vi "超标留样通讯.vi"(8 "error in (no error)":errorcluster, 9 "VISA resource name":refnum<visa-resource-name> caption="VISA资源名称", 10 "写入缓冲区":string, 11 "功能输入":enum16{"打开串口", "写入", "读取", "关闭串口"}(ring)) -> (0 "error out":errorcluster, 2 "读取缓冲区":string, 3 "VISA resource name out":refnum<visa-resource-name>)   [LabVIEW 2016, in "超标留样集成.lvlib" / "德润DR803M超标留样.lvlib"]
uses:
  <vilib>/Instr/_visa.llb/VISA Configure Serial Port (Instr).vi
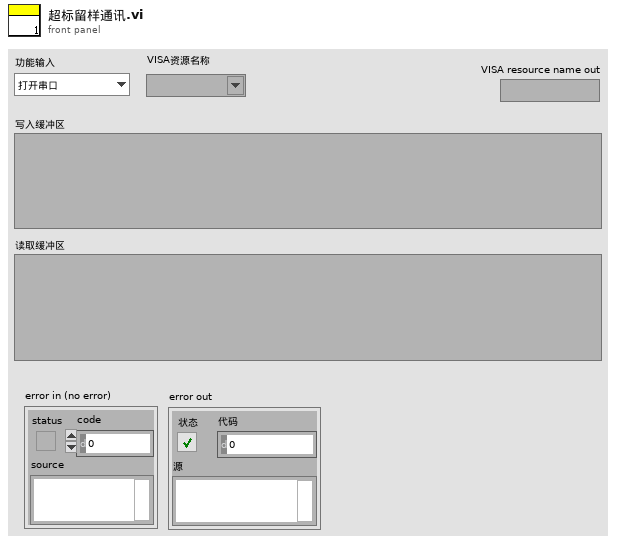
[diagram p1: front panel]
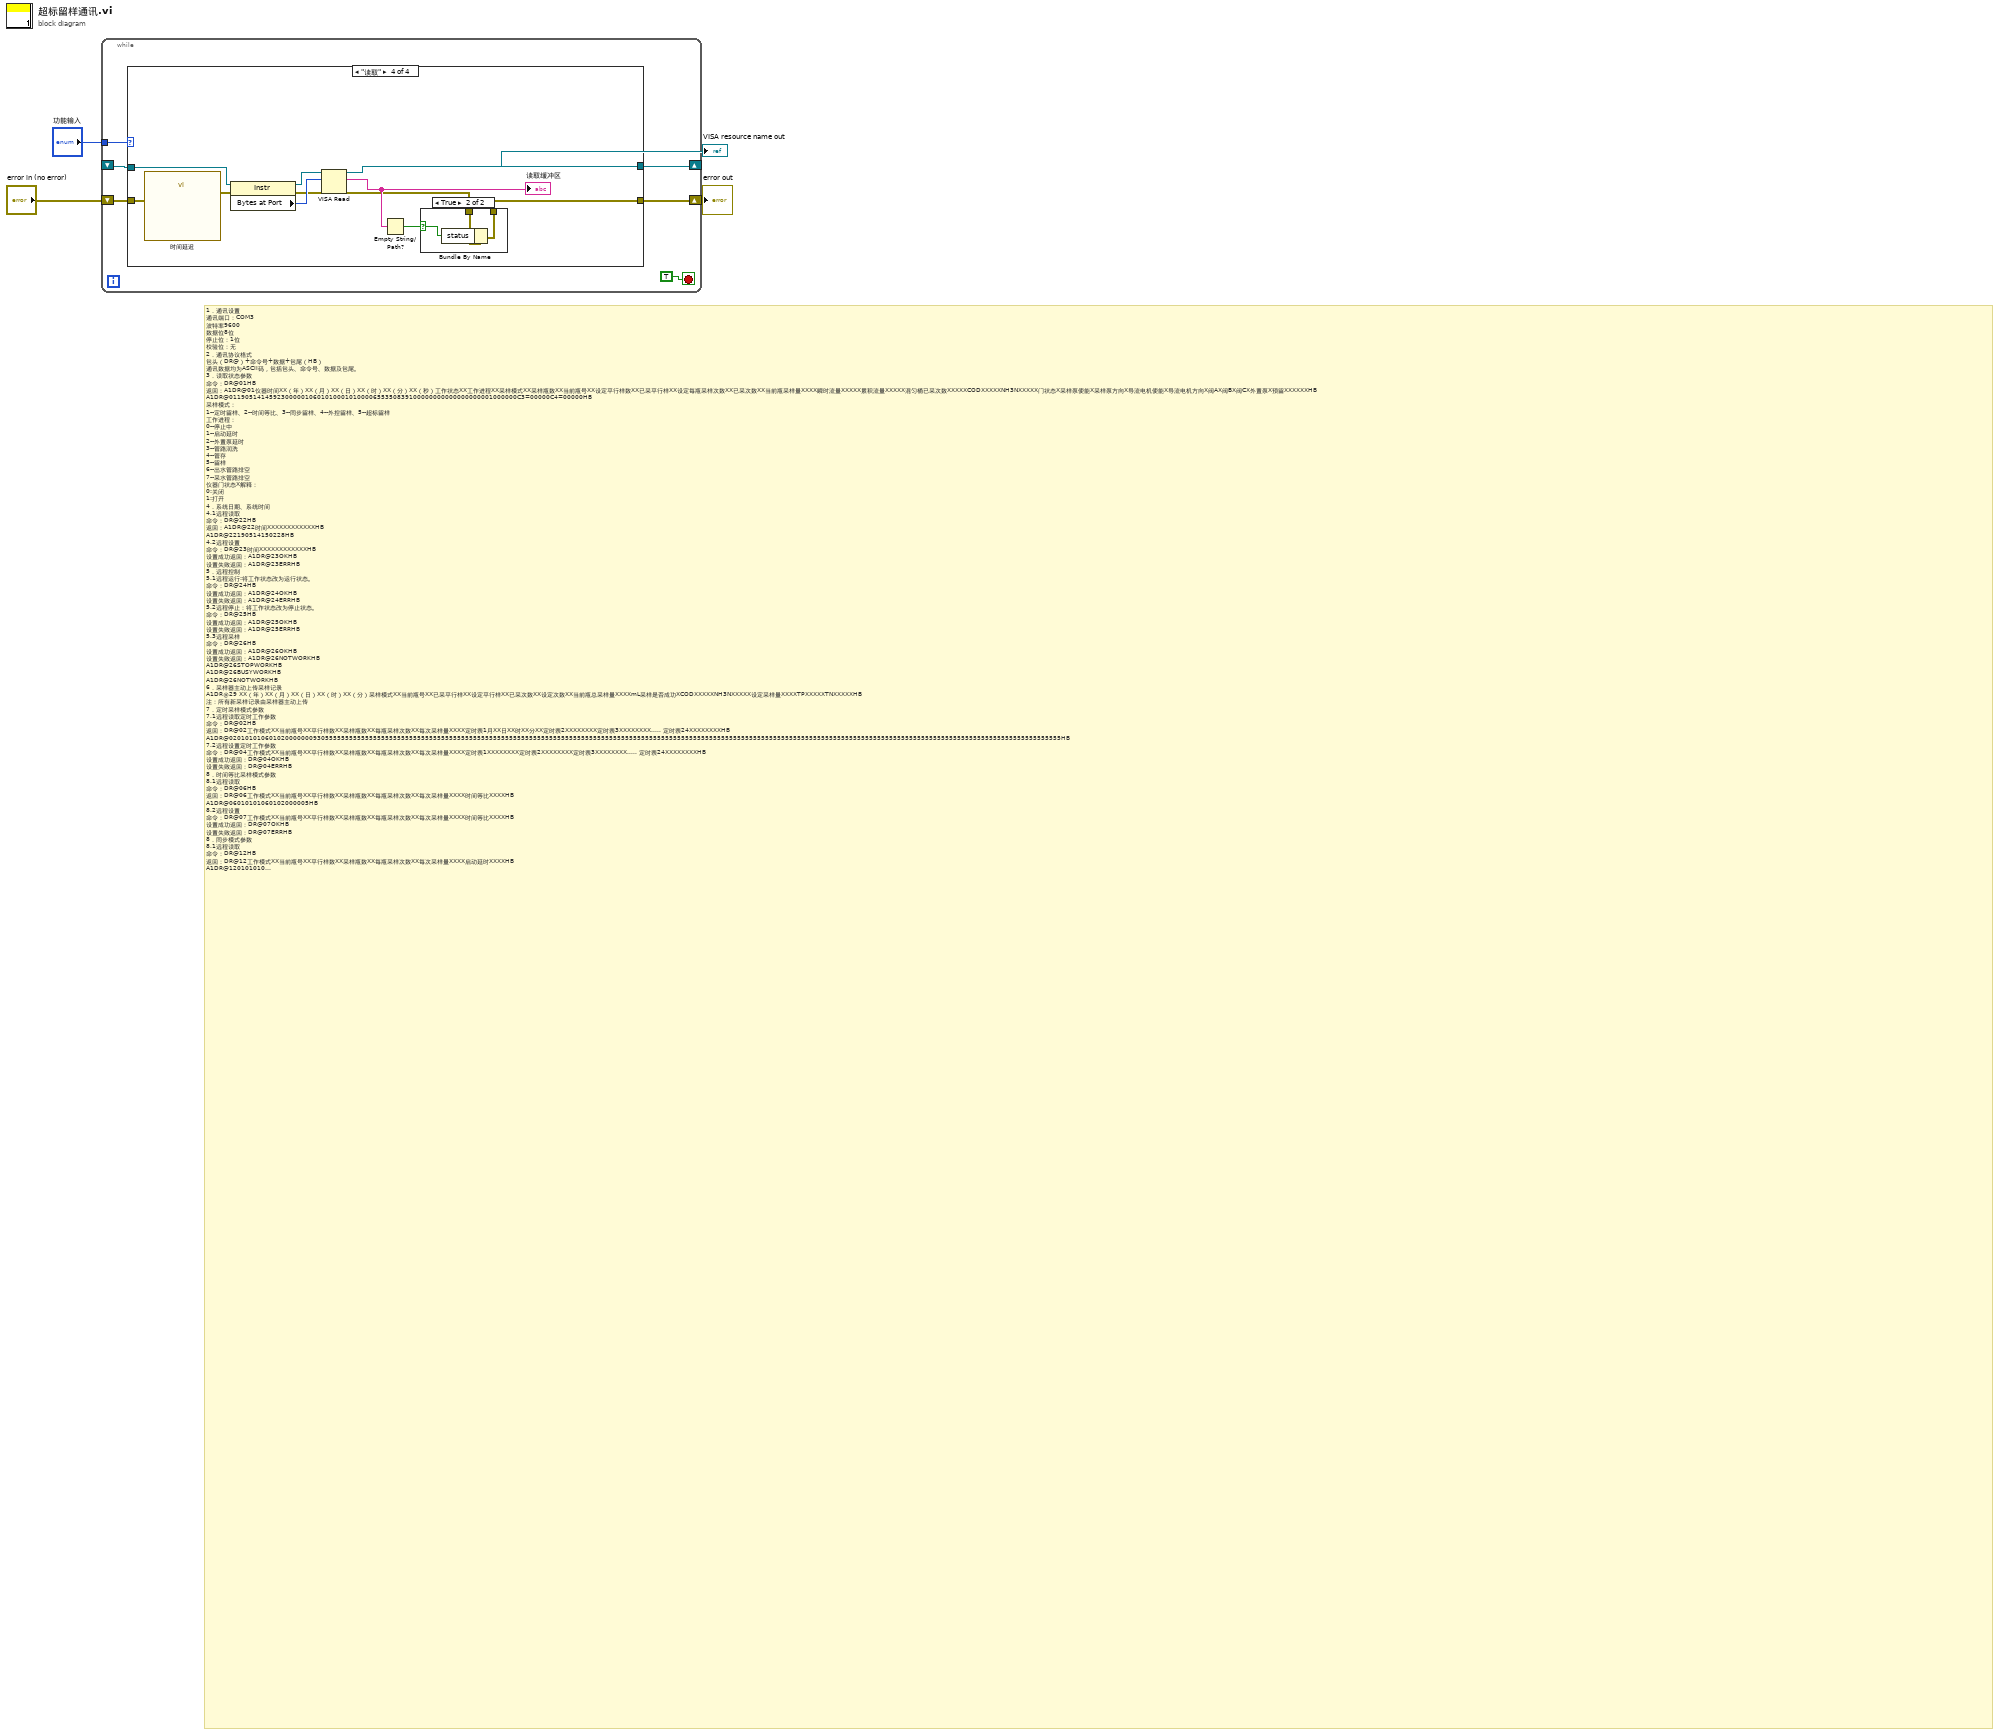
[diagram p0: block diagram]
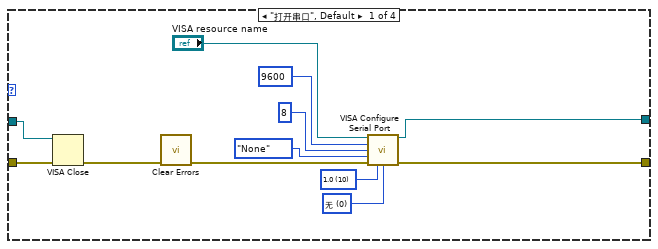
[diagram p2: hidden frame]
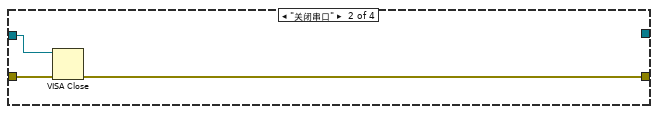
[diagram p3: hidden frame]
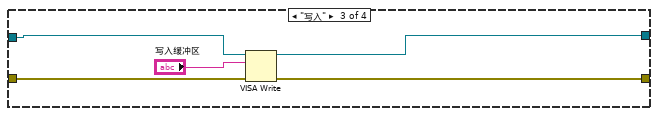
[diagram p4: hidden frame]
diagram:
  # "1．通讯设置\n通讯端口：COM3\n波特率9600 \n数据位8位\n停止位：1位\n校验位：无\n2．通讯协议格式\n包头（DR@）+命令号+数据+包尾（HB）\n通讯数据均为ASCII码，包括包头、命令号、数据及包尾。\n3．读取状态参数\n命令：DR@01HB\n返回：A1DR@01仪器时间XX（年）XX（月）XX（日）XX（时）XX（分）XX（秒）工作状态XX工作进程XX采样模式XX采样瓶数XX当前瓶号XX设定平行样数XX已采平行样XX设定每瓶采样次数XX已采次数XX当前瓶采样量XXXX瞬时流量XXXXX累积流量XXXXX混匀桶已采次数XXXXXCODXXXXXNH3NXXXXX门状态X采样泵使能X采样泵方向X导流电机使能X导流电机方向X阀AX阀BX阀CX外置泵X预留XXXXXXHB\nA1DR@011905141459230000010601010001010000655350839100000000000000000001000000C3=00000C4=00000HB\n采样模式：\n1--定时留样、2--时间等比、3--同步留样、4--外控留样、5--超标留样\n工作进程：\n0--停止中\n1--启动延时\n2--外置泵延时\n3--管路润洗\n4--管存\n5--留样\n6--出水管路排空\n7--采水管路排空\n仪器门状态X解释：\n0:关闭\n1:打开\n4．系统日期、系统时间\n4.1远程读取 \n命令：DR@22HB\n返回：A1DR@22时间XXXXXXXXXXXXHB\nA1DR@22190514150228HB\n4.2远程设置\n命令：DR@23时间XXXXXXXXXXXXHB\n设置成功返回：A1DR@23OKHB\n设置失败返回：A1DR@23ERRHB\n5．远程控制\n5.1远程运行:将工作状态改为运行状态。\n命令：DR@24HB\n设置成功返回：A1DR@24OKHB\n设置失败返回：A1DR@24ERRHB\n5.2远程停止：将工作状态改为停止状态。\n命令：DR@25HB\n设置成功返回：A1DR@25OKHB\n设置失败返回：A1DR@25ERRHB\n5.3远程采样\n命令：DR@26HB\n设置成功返回：A1DR@26OKHB\n设置失败返回：A1DR@26NOTWORKHB\nA1DR@26STOPWORKHB\nA1DR@26BUSYWORKHB\nA1DR@26NOTWORKHB\n6．采样器主动上传采样记录\nA1DR＠29 XX（年）XX（月）XX（日）XX（时）XX（分）采样模式XX当前瓶号XX已采平行样XX设定平行样XX已采次数XX设定次数XX当前瓶总采样量XXXXmL采样是否成功XCODXXXXXNH3NXXXXX设定采样量XXXXTPXXXXXTNXXXXXHB\n注：所有新采样记录由采样器主动上传\n7．定时采样模式参数\n7.1远程读取定时工作参数\n命令：DR@02HB\n返回：DR@02工作模式XX当前瓶号XX平行样数XX采样瓶数XX每瓶采样次数XX每次采样量XXXX定时表1月XX日XX时XX分XX定时表2XXXXXXXX定时表3XXXXXXXX..... 定时表24XXXXXXXXHB\nA1DR@0201010106010200000009305555555555555555555555555555555555555555555555555555555555555555555555555555555555555555555555555555555555555555555555555555555555555555555555555555555555555555555555555555555555555555HB\n7.2远程设置定时工作参数\n命令：DR@04工作模式XX当前瓶号XX平行样数XX采样瓶数XX每瓶采样次数XX每次采样量XXXX定时表1XXXXXXXX定时表2XXXXXXXX定时表3XXXXXXXX..... 定时表24XXXXXXXXHB\n设置成功返回：DR@04OKHB\n设置失败返回：DR@04ERRHB\n8．时间等比采样模式参数\n8.1远程读取\n命令：DR@06HB\n返回：DR@06工作模式XX当前瓶号XX平行样数XX采样瓶数XX每瓶采样次数XX每次采样量XXXX时间等比XXXXHB\nA1DR@06010101060102000005HB\n8.2远程设置\n命令：DR@07工作模式XX当前瓶号XX平行样数XX采样瓶数XX每瓶采样次数XX每次采样量XXXX时间等比XXXXHB\n设置成功返回：DR@07OKHB\n设置失败返回：DR@07ERRHB\n8．同步模式参数\n8.1远程读取\n命令：DR@12HB\n返回：DR@12工作模式XX当前瓶号XX平行样数XX采样瓶数XX每瓶采样次数XX每次采样量XXXX启动延时XXXXHB\nA1DR@12010101060102000010HB\n8.2远程设置\n命令：DR@13工作模式XX当前瓶号XX平行样数XX采样瓶数XX每瓶采样次数XX每次采样量XXXX启动延时XXXXHB\n设置成功返回：DR@13OKHB\n设置失败返回：DR@13ERRHB\n9. 外控留样模式参数\n9.1远程读取\n命令：DR@58HB\n返回：DR@58工作模式XX当前瓶号XX平行样数XX采样瓶数XX每瓶采样次数XX每次采样量XXXXHB\nA1DR@5801010106010200HB\n9.2远程设置\nDR@59工作模式XX当前瓶号XX平行样数XX采样瓶数XX每瓶采样次数XX每次采样量XXXXHB\n设置成功返回：DR@59OKHB\n设置失败返回：DR@59ERRHB\n10．超标模式参数\n10.1远程读取\n命令：DR@16\n返回：DR@16工作模式XX当前瓶号XX平行样数XX采样瓶数XX每瓶采样次数XX每次采样量XXXX采样间隔时间XXXXCOD联机方式XX4mA浓度XXXXX 20mA浓度XXXXX超标浓度XXXXX当前浓度浓度XXXXX NH3N联机方式XX4mA浓度XXXXX 20mA浓度XXXXX超标浓度XXXXX当前浓度浓度XXXXXHB\nA1DR@1605010106010200000503000001000001000000000300000010000010000000HB\n10.2远程设置\n命令：DR@17工作模式XX当前瓶号XX平行样数XX采样瓶数XX每瓶采样次数XX每次采样量XXXX采样间隔XXXXCOD联机方式XX NH3N联机方式XX  COD4mA浓度XXXXX 20mA浓度XXXXX超标浓度XXXXX NH3N 4mA浓度XXXXX 20mA浓度XXXXX超标浓度XXXXX HB\n设置成功返回：DR@17OKHB\n设置失败返回：DR@17ERRHB"
  n1 = while {
    shift-right: [w9] -> w1
    shift-left: _ -> [w7]
    shift-right: [w8] -> w2
    shift-left: "error in (no error)" -> [w6]
    tunnel: "功能输入" -> [w5]
    stop <- TRUE stop-if-true
    n2 = case shown="\"读取\"" w5 {
      tunnel: [w13 _ w28 w40] -> w9
      tunnel: [w12 w25 w27 w32] -> w8
      tunnel: w7 -> [w21 w24 w30 w39]
      tunnel: w6 -> [w22 w23 w29 w41]
      frame "打开串口", Default {
        w14 = u16 0 items=["无", "XON/XOFF", "RTS/CTS", "XON/XOFF & RTS/CTS", "DTR/DSR", "XON/XOFF & DTR/DSR"] ("flow control (0:none)")
        w16 = u16 10 items=["1.0"=10, "1.5"=15, "2.0"=20] ("stop bits (10: 1 bit)")
        n3 = VISA Close(VISA resource name=w21, error in (no error)=w22) -> (error out=w20:errorcluster)
        n4 = call <vilib>:"Clear Errors.vi"("error in (no error)"=w20) -> ("error out"=w19:errorcluster)  [unwired: 5 in, 1 out]
        n5 = call-poly "VISA Configure Serial Port"("VISA resource name"="VISA resource name", "baud rate (9600)"=u32 9600, "data bits (8)"=u16 8, "parity (0:none)"=enum16{"None", "Odd", "Even", "Mark", "Space"}."None", "error in (no error)"=w19, "stop bits (10: 1 bit)"=w16, "flow control (0:none)"=w14) -> ("VISA resource name out"=w13:refnum<visa-resource-name>, "error out"=w12:errorcluster)  [unwired: 7 in]
      }
      frame "关闭串口" {
        n6 = VISA Close(VISA resource name=w24, error in (no error)=w23) -> (error out=w25:errorcluster)
      }
      frame "写入" {
        n7 = VISA Write(VISA resource name=w30, write buffer="写入缓冲区", error in (no error)=w29) -> (VISA resource name out=w28:refnum<visa-resource-name>, error out=w27:errorcluster)  [unwired: 1 out]
      }
      frame "读取" {
        n8 = call "时间延迟"("error in (no error)"=w41) -> ("error out"=w37:errorcluster)  [unwired: 10 in]
        n9 = property class="Instr"(reference=w39, error in=w37) -> (reference out=w35:refnum<visa-resource-name>, error out=w36:errorcluster, "Bytes at Port"=w38:u32)
        n10 = VISA Read(VISA resource name=w35, byte count=w38, error in (no error)=w36) -> (VISA resource name out=w40:refnum<visa-resource-name>, read buffer=w34:string, error out=w31:errorcluster)  [unwired: 1 out]
        "读取缓冲区" <- w34
        n11 = Empty String/Path?(string/path=w34) -> (empty?=w33:bool)
        n12 = case shown="True" w33 {
          selector: w33 -> [_ w43]
          tunnel: w31 -> [w42 w45]
          tunnel: [w42 w44] -> w32
          frame False {
          }
          frame True {
            n13 = Bundle By Name(cluster=w45, "status"=w43) -> (w44:errorcluster)
          }
        }
      }
    }
  }
  "error out" <- w2
  "VISA resource name out" <- w1
